vi "Orca Flash Fix ROI Size.vi"(0 "Requested Value 1":i32, 2 "Allowed Increment":i32, 5 "Requested Value 2":i32, 7 "Requested Value 3":i32, 9 "Requested Value 4":i32) -> (4 "Resulting Value 1":i32, 6 "Resulting Value 2":i32, 8 "Resulting Value 3":i32, 10 "Resulting Value 4":i32)   [LabVIEW 2025]
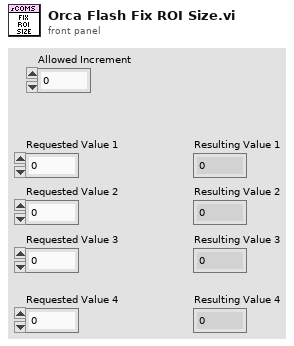
[diagram p1: front panel]
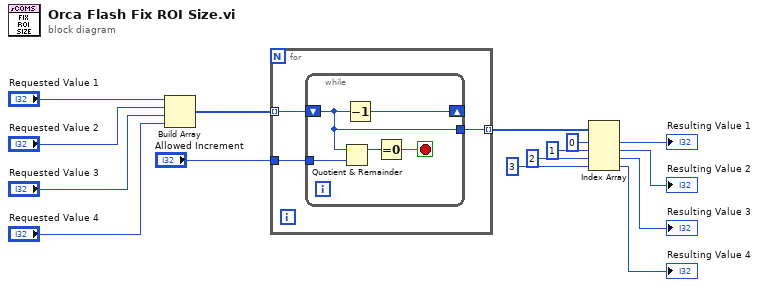
[diagram p0: block diagram]
diagram:
  n1 = Build Array("Requested Value 1", "Requested Value 2", "Requested Value 3", "Requested Value 4") -> (w10:i32[])
  n2 = for {
    tunnel: "Allowed Increment" -> [w18]
    tunnel: w10 -> [w17] mode=indexing
    tunnel: [w16] -> w9 mode=indexing
    n3 = while {
      shift-right: [w21] -> _
      shift-left: w17 -> [w20]
      tunnel: [w20] -> w16
      tunnel: w18 -> [w19]
      stop <- w22 stop-if-true
      n4 = Quotient & Remainder(x=w20, y=w19) -> (x-y*floor(x/y)=w23:i32)  [unwired: 1 out]
      n5 = Decrement(x=w20) -> (x-1=w21:i32)
      n6 = Equal To 0?(x=w23) -> (x = 0?=w22:bool)
    }
  }
  n7 = Index Array(array=w9, index #1=0 ("index"), index #2=1 ("index"), index #3=2 ("index"), index #4=3 ("index")) -> (element #1=→"Resulting Value 1":i32, element #2=→"Resulting Value 2":i32, element #3=→"Resulting Value 3":i32, element #4=→"Resulting Value 4":i32)
